vi "codigo.vi"() -> ()   [LabVIEW 2020]
uses:
  Pos_modifi.vi
  Llenado.vi
  Pos_iniciales.vi
  Pos_iniciales1.vi
  Pos_iniciales3.vi
  sensores.vi
panel:
  in  "PistonC":bool
  in  "PistonA":bool
  in  "Laminadora":bool
  in  "Sensor 1":bool
  in  "Llenado":T1 {"Mezclador" scale=0.0..10.0; "Pintado" scale=0.0..10.0; "Tanque" scale=0.0..100.0; "Llenador" scale=0.0..100.0; "Bote" scale=0.0..100.0}
  in  "Pos_modif":T2
  out "Pos_Iniciales3":T3
  out "Pos_Iniciales1":T4
  out "Pos_Iniciales":T5
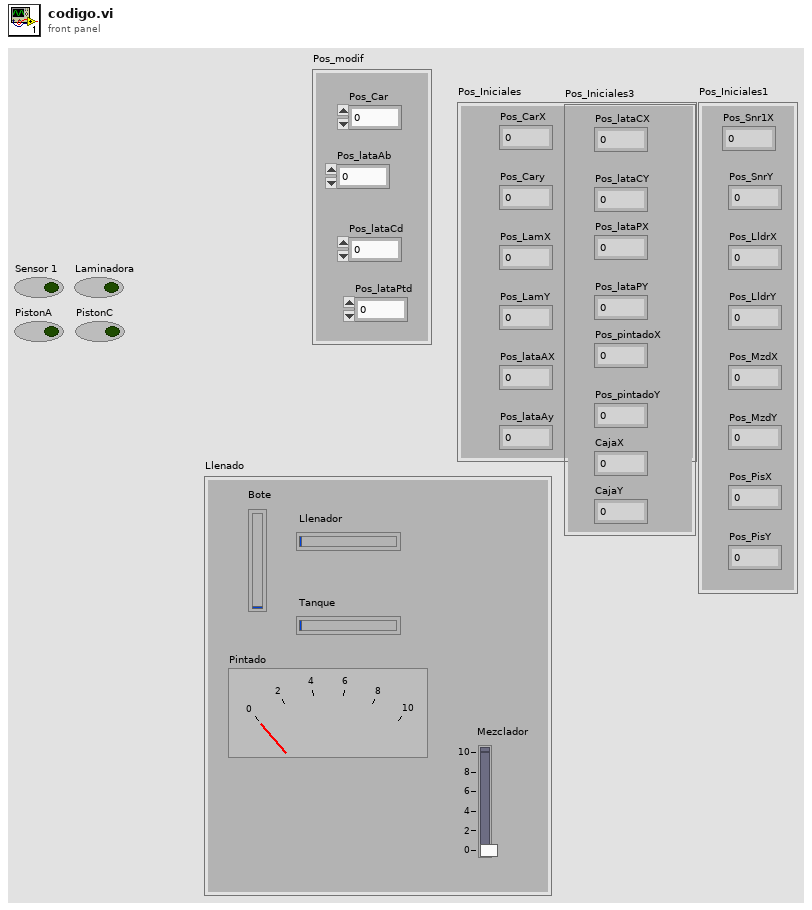
[diagram p1: front panel]
types:
  T1 = cluster{"Bote":u8, "Llenador":u8, "Tanque":u8, "Pintado":dbl, "Mezclador":dbl}
  T2 = cluster{"Pos_Car":dbl, "Pos_lataAb":dbl, "Pos_lataCd":dbl, "Pos_lataPtd":dbl}
  T3 = cluster{"Pos_lataCX":dbl, "Pos_lataCY":dbl, "Pos_lataPX":dbl, "Pos_lataPY":dbl, "Pos_pintadoX":dbl, "Pos_pintadoY":dbl, "CajaX":dbl, "CajaY":dbl}
  T4 = cluster{"Pos_Snr1X":dbl, "Pos_SnrY":dbl, "Pos_LldrX":dbl, "Pos_LldrY":dbl, "Pos_MzdX":dbl, "Pos_MzdY":dbl, "Pos_PisX":dbl, "Pos_PisY":dbl}
  T5 = cluster{"Pos_CarX":dbl, "Pos_Cary":dbl, "Pos_LamX":dbl, "Pos_LamY":dbl, "Pos_lataAX":dbl, "Pos_lataAy":dbl}
  T6 = cluster{"Sensor 1":bool, "Laminadora":bool, "PistonA":bool, "PistonC":bool}
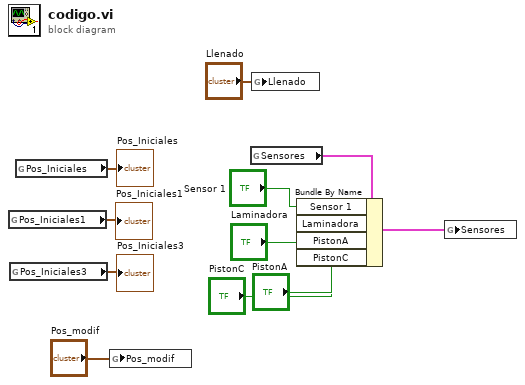
[diagram p0: block diagram]
diagram:
  n1 = global read "Pos_iniciales1.vi" "Pos_Iniciales1"() -> (→"Pos_Iniciales1":T4)
  n2 = global read "Pos_iniciales3.vi" "Pos_Iniciales3"() -> (→"Pos_Iniciales3":T3)
  n3 = global read "Pos_iniciales.vi" "Pos_Iniciales"() -> (→"Pos_Iniciales":T5)
  n4 = global write "Pos_modifi.vi" "Pos_modif"("Pos_modif") -> ()
  n5 = global read "sensores.vi" "Sensores"() -> (w6:T6)
  n6 = global write "Llenado.vi" "Llenado"("Llenado") -> ()
  n7 = Bundle By Name(cluster=w6, "Sensor 1"="Sensor 1", "Laminadora"="Laminadora", "PistonA"="PistonA", "PistonC"="PistonC") -> (w5:T6)
  n8 = global write "sensores.vi" "Sensores"(w5) -> ()
